vi "Anritsu VNA Convert Formated Data.vi"(7 "Display Format":T1, 10 "Number":cdb) -> (2 "Number":cdb)   [LabVIEW 2011]
uses:
  tests/S Parameter/TypeDefs/SP Measurement Format.ctl
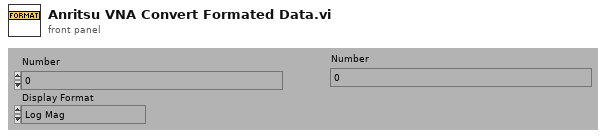
[diagram p1: front panel]
types:
  T1 = typedef "SP Measurement Format.ctl" = enum32{"Log Mag", "Phase", "Delay", "Smith (R+jX)", "Polar (Re/Im)", "Linear Mag", "SWR", "Real", "Imaginary", "Smith (Lin/Phase)", "Smith (Log/Phase)", "Smith (Real/Imag)", "Smith (G+jB)", "Polar (Lin/Phase)", "Polar (Log/Phase)", "Expanded Phase", "Positive Phase", "Inverted Smith", "Unwrapped Phase", "Power Out", "Power In", "Linear Mag/Phase", "Log Mag/Phase", "Real/Imaginary"}
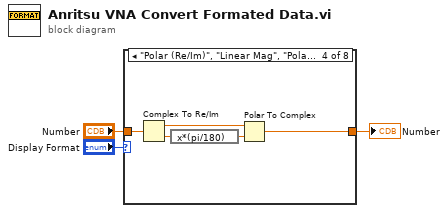
[diagram p0: block diagram]
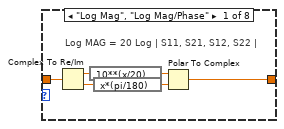
[diagram p2: hidden frame]
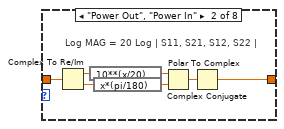
[diagram p3: hidden frame]
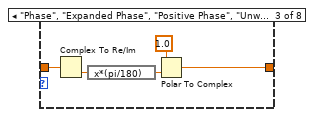
[diagram p4: hidden frame]
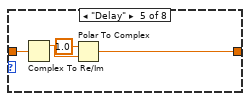
[diagram p5: hidden frame]
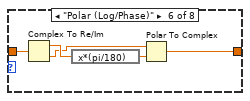
[diagram p6: hidden frame]
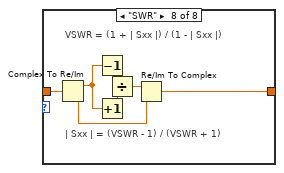
[diagram p8: hidden frame]
diagram:
  n1 = case shown="\"Polar (Re/Im)\", \"Linear Mag\", \"Polar (Lin/Phase)\", \"Linear Mag/Phase\"" "Display Format" {
    tunnel: [w4 w10 w20 w23 w27 w33 w36 w40] -> w2
    tunnel: "Number" -> [w8 w15 w21 w24 w28 w35 w36 w41]
    frame "Log Mag", "Log Mag/Phase" {
      # "Log MAG = 20 Log | S11, S21, S12, S22 |"
      n2 = Complex To Re/Im(x + iy=w8) -> (x=w9:dbl, y=w7:dbl)
      n3 = expression code="10**(x/20)"(w9) -> (w6:dbl)
      n4 = expression code="x*(pi/180)"(w7) -> (w5:dbl)
      n5 = Polar To Complex(1:w5, 2:w6) -> (0:w4:cdb)
    }
    frame "Power Out", "Power In" {
      # "Log MAG = 20 Log | S11, S21, S12, S22 |"
      n6 = Complex To Re/Im(x + iy=w15) -> (x=w16:dbl, y=w14:dbl)
      n7 = expression code="10**(x/20)"(w16) -> (w13:dbl)
      n8 = expression code="x*(pi/180)"(w14) -> (w12:dbl)
      n9 = Polar To Complex(1:w12, 2:w13) -> (0:w11:cdb)
      n10 = Complex Conjugate(1:w11) -> (0:w10:cdb)
    }
    frame "Phase", "Expanded Phase", "Positive Phase", "Unwrapped Phase" {
      n11 = Complex To Re/Im(x + iy=w21) -> (y=w19:dbl)  [unwired: 1 out]
      n12 = expression code="x*(pi/180)"(w19) -> (w18:dbl)
      n13 = Polar To Complex(1:w18, 2:1.0 ("r")) -> (0:w20:cdb)
    }
    frame "Polar (Re/Im)", "Linear Mag", "Polar (Lin/Phase)", "Linear Mag/Phase" {
      n14 = Complex To Re/Im(x + iy=w24) -> (x=w22:dbl, y=w26:dbl)
      n15 = expression code="x*(pi/180)"(w26) -> (w25:dbl)
      n16 = Polar To Complex(1:w25, 2:w22) -> (0:w23:cdb)
    }
    frame "Delay" {
      n17 = Complex To Re/Im(x + iy=w28) -> (x=w29:dbl)  [unwired: 1 out]
      n18 = Polar To Complex(1:w29, 2:1.0 ("r")) -> (0:w27:cdb)
    }
    frame "Polar (Log/Phase)" {
      n19 = Complex To Re/Im(x + iy=w35) -> (x=w32:dbl, y=w31:dbl)
      n20 = expression code="x*(pi/180)"(w32) -> (w34:dbl)
      n21 = Polar To Complex(1:w34, 2:w31) -> (0:w33:cdb)
    }
    frame "Smith (R+jX)", "Real".."Smith (G+jB)", "Inverted Smith", "Real/Imaginary" {
    }
    frame "SWR" {
      # "| Sxx | = (VSWR - 1) / (VSWR + 1)"
      # "VSWR = (1 + | Sxx |) / (1 - | Sxx |)"
      n22 = Complex To Re/Im(x + iy=w41) -> (x=w38:dbl, y=w37:dbl)
      n23 = Decrement(x=w38) -> (x-1=w43:dbl)
      n24 = Increment(x=w38) -> (x+1=w42:dbl)
      n25 = Divide(x=w43, y=w42) -> (x/y=w39:dbl)
      n26 = Re/Im To Complex(1:w37, 2:w39) -> (0:w40:cdb)
    }
  }
  "Number" <- w2
